vi "zmq_REP_server.vi"() -> ()   [LabVIEW 2012]
doc: "Sends a specified waveform through a TCP port. The VI first listens for a connection and, once established, sends the number of bytes to be sent followed by the data. After the data is sent, the VI waits for an 'all received' signal from the client and then breaks the connection.\n\n<B>Note:</B> Requires the Data Client.vi located in the same library as this VI."
uses:
  <vilib>/addons/zeromq/socket_type.ctl
panel:
  in  "amplitude period (ms)":u32=1000
  out "Waveform Graph":dbl[](graph)=[nan, nan, nan, nan, nan, nan, nan, nan, nan, nan, nan, nan, nan, nan, nan, nan, nan, nan, nan, nan, nan, nan, nan, nan, nan, nan, nan, nan, nan, nan, nan, nan, nan, nan, nan, nan, nan, nan, nan, nan, nan, nan, nan, nan, nan, nan, nan, nan, nan, nan, nan, nan, nan, nan, nan, nan, nan, nan, nan, nan, nan, nan, nan, nan, nan, nan, nan, nan, nan, nan, nan, nan, nan, nan, nan, nan, nan, nan, nan, nan, nan, nan, nan, nan, nan, nan, nan, nan, nan, nan, nan, nan, nan, nan, nan, nan, nan, nan, nan, nan, nan, nan, nan, nan, nan, nan, nan, nan, nan, nan, nan, nan, nan, nan, nan, nan, nan, nan, nan, nan, nan, nan, nan, nan, nan, nan, nan, nan, nan, nan, nan, nan, nan, nan, nan, nan, nan, nan, nan, nan, nan, nan, nan, nan, nan, nan, nan, nan, nan, nan, nan, nan, nan, nan, nan, nan, nan, nan, nan, nan, nan, nan, nan, nan, nan, nan, nan, nan, nan, nan, nan, nan, nan, nan, nan, nan, nan, nan, nan, nan, nan, nan, nan, nan, nan, nan, nan, nan, nan, nan, nan, nan, nan, nan, nan, nan, nan, nan, nan, nan]
  in  "stop":bool
  in  "Noise Level":dbl(slide)=0.36734693877551017 scale=0.0..1.0 scale format="%0.1f"
  in  "# of Points":i32=200
  in  "Function":u16(ring)=2 items=["random", "sine wave", "cosine wave"]
  in  "Port":u16=6340 min=1025 step=1
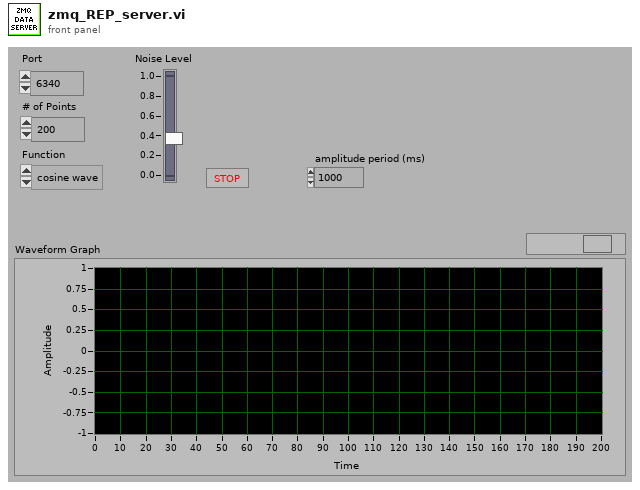
[diagram p1: front panel]
types:
  T1 = typedef "zeromq.lvlib/socket_type.ctl" = enum8{"ZMQ_PAIR", "ZMQ_PUB", "ZMQ_SUB", "ZMQ_REQ", "ZMQ_REP", "ZMQ_DEALER", "ZMQ_ROUTER", "ZMQ_PULL", "ZMQ_PUSH", "ZMQ_XPUB", "ZMQ_XSUB"}
  T2 = typedef "pointer.ctl" = u64
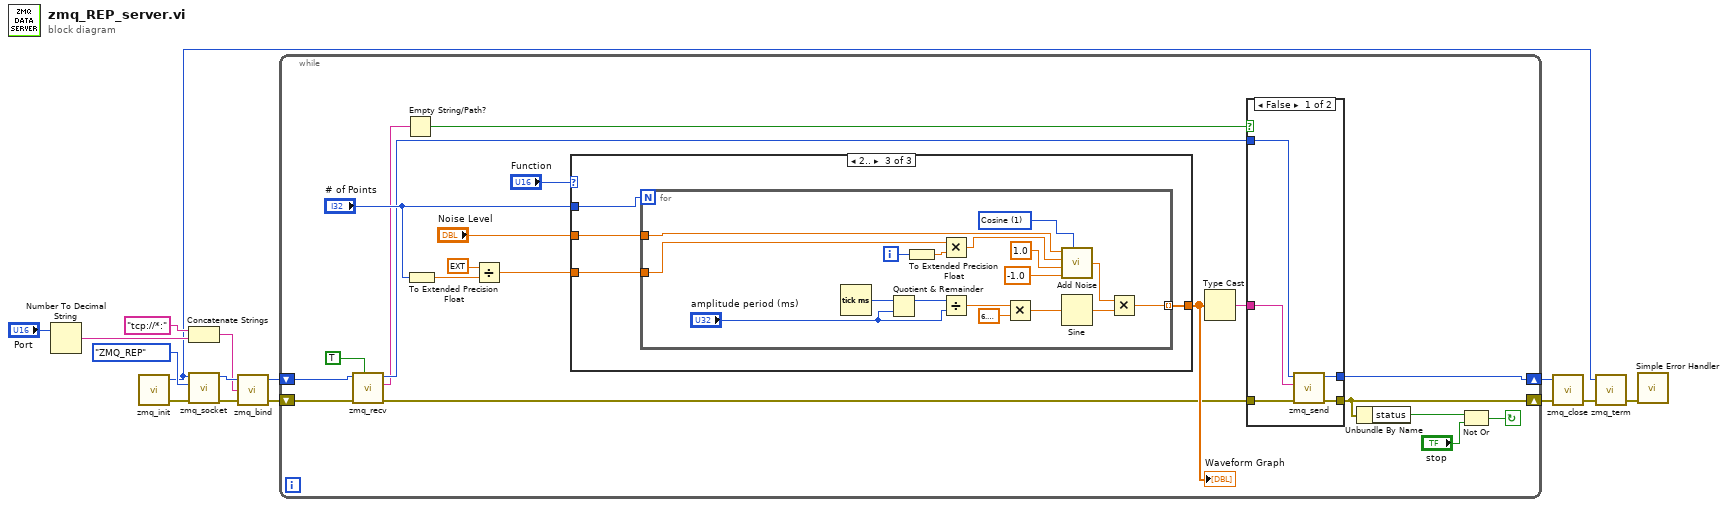
[diagram p0: block diagram]
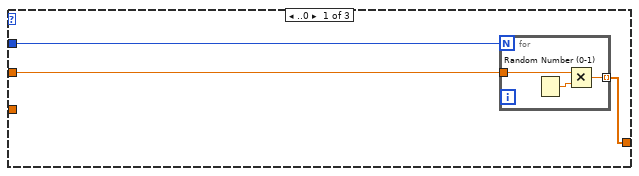
[diagram p3: hidden frame]
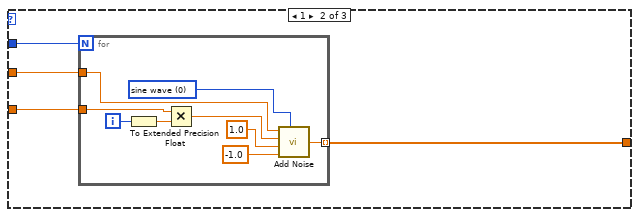
[diagram p4: hidden frame]
diagram:
  n1 = Number To Decimal String(number="Port") -> (decimal integer string=w8:string)  [unwired: 1 in]
  n2 = call <vilib>:"zmq_init.vi"() -> ("error out"=w14:errorcluster, "context"=w1:T2)  [unwired: 4 in]
  n3 = Concatenate Strings("tcp://*:" ("port"), w8) -> (w10:string)
  n4 = call <vilib>:"zmq_socket.vi"("error in"=w14, "socket type"=socket_type."ZMQ_REP", "ctx in"=w1) -> ("error out"=w13:errorcluster, "socket"=w12:T2)  [unwired: 3 in]
  n5 = call <vilib>:"zmq_bind.vi"("error in"=w13, "endpoint"=w10, "socket in"=w12) -> ("error out"=w4:errorcluster, "socket out"=w3:T2)  [unwired: 1 in]
  n6 = while {
    shift-right: [w23] -> w2
    shift-left: w3 -> [w22]
    shift-right: [w25] -> w5
    shift-left: w4 -> [w20]
    stop <- w35 continue-if-true
    n7 = call <vilib>:"zmq_recv.vi"("no block? (F)"=TRUE, "error in"=w20, "socket in"=w22) -> ("error out"=w19:errorcluster, "data"=w17:string, "socket out"=w21:T2)  [unwired: 2 in, 2 out]
    n8 = Empty String/Path?(string/path=w17) -> (empty?=w16:bool)
    n9 = To Extended Precision Float(1:"# of Points") -> (0:w33:ext)
    n10 = Divide(x=ext 6.283185307179586477, y=w33) -> (x/y=w30:ext)
    n11 = case shown="2.." "Function" {
      tunnel: "# of Points" -> [w45 w52 w65]
      tunnel: [w44 w49 w62] -> w27
      tunnel: w30 -> [_ w51 w63]
      tunnel: "Noise Level" -> [w43 w50 w64]
      frame ..0 {
        n12 = for {
          N: w45 -> [_]
          tunnel: [w46] -> w44 mode=indexing
          tunnel: w43 -> [w48]
          n13 = Random Number (0-1)() -> (number: 0 to 1=w47:dbl)
          n14 = Multiply(x=w48, y=w47) -> (x*y=w46:dbl)
        }
      }
      frame 1 {
        n15 = for {
          N: w52 -> [_]
          tunnel: w51 -> [w60]
          tunnel: w50 -> [w59]
          tunnel: [w58] -> w49 mode=indexing
          i -> [w61]
          w53 = u16 0 items=["sine wave", "cosine wave"] ("Function")
          n16 = To Extended Precision Float(1:w61) -> (0:w57:ext)
          n17 = Multiply(x=w60, y=w57) -> (x*y=w54:ext)
          n18 = call "Add Noise.vi"("noise"=w59, "input"=w54, "max"=1.0, "min"=-1.0, "Function"=w53) -> ("output"=w58:dbl)
        }
      }
      frame 2.. {
        n19 = for {
          N: w65 -> [_]
          tunnel: w64 -> [w78]
          tunnel: w63 -> [w77]
          tunnel: [w70] -> w62 mode=indexing
          i -> [w82]
          w75 = u16 1 items=["Sine", "Cosine"] ("Function")
          n20 = Tick Count (ms)() -> (millisecond timer value=w74:u32)
          n21 = Quotient & Remainder(x=w74, y="amplitude period (ms)") -> (x-y*floor(x/y)=w73:u32)  [unwired: 1 out]
          n22 = To Extended Precision Float(1:w82) -> (0:w81:ext)
          n23 = Multiply(x=w77, y=w81) -> (x*y=w76:ext)
          n24 = Divide(x=w73, y="amplitude period (ms)") -> (x/y=w69:dbl)
          n25 = Multiply(x=w69, y=6.283185307179586) -> (x*y=w67:dbl)
          n26 = call "Add Noise.vi"("noise"=w78, "input"=w76, "max"=1.0, "min"=-1.0, "Function"=w75) -> ("output"=w71:dbl)
          n27 = Sine(x=w67) -> (sin(x)=w66:dbl)
          n28 = Multiply(x=w71, y=w66) -> (x*y=w70:dbl)
        }
      }
    }
    "Waveform Graph" <- w27
    n29 = Type Cast(x=w27) -> (*(type *) &x=w26:string)  [unwired: 1 in]
    n30 = case shown="False" w16 {
      tunnel: w26 -> [w40 _]
      tunnel: [w39 w42] -> w25
      tunnel: [w38 w41] -> w23
      tunnel: w21 -> [w37 w41]
      tunnel: w19 -> [w36 w42]
      frame False {
        n31 = call <vilib>:"zmq_send.vi"("error in"=w36, "data"=w40, "socket in"=w37) -> ("error out"=w39:errorcluster, "socket out"=w38:T2)  [unwired: 4 in]
      }
      frame True {
      }
    }
    n32 = Unbundle By Name(w25) -> ("status"=w34:bool)
    n33 = Not Or(1:"stop", 2:w34) -> (0:w35:bool)
  }
  n34 = call <vilib>:"zmq_close.vi"("error in"=w5, "socket in"=w2) -> ("error out"=w7:errorcluster)  [unwired: 3 in]
  n35 = call <vilib>:"zmq_term.vi"("error in"=w7, "context"=w1) -> ("error out"=w6:errorcluster)  [unwired: 3 in]
  n36 = call <vilib>:"Simple Error Handler.vi"("error in (no error)"=w6) -> ()  [unwired: 4 in, 5 out]
